vi "Enqueue Message.vi"(6 "Priority Message? (F)":bool=TRUE, 8 "error in (no error)":errorcluster, 10 "Message":T1={"Source"="", "Destination"="", "Time Stamp"=timestamp(0 s since 1904-01-01), "Command"="", "Data"=variant(string "")}, 11 "Listening Queue":refnum<queue>) -> (0 "error out":errorcluster, 3 "queue out":refnum<queue>)   [LabVIEW 2018, in "Dynamic Reentrant.lvlib"]
uses:
  <userlib>/Dynamic Reentrant/Dynamic Reentrant.lvlib
  <userlib>/Dynamic Reentrant/Type Defs/Message.ctl
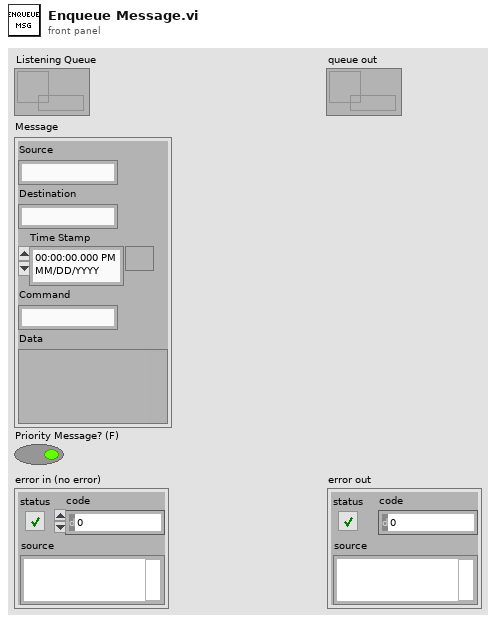
[diagram p1: front panel]
types:
  T1 = typedef "Dynamic Reentrant.lvlib/Message.ctl" = cluster{"Source":string, "Destination":string, "Time Stamp":timestamp, "Command":string, "Data":variant}
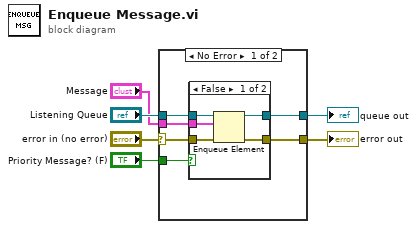
[diagram p0: block diagram]
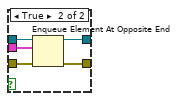
[diagram p2: hidden frame]
diagram:
  n1 = case shown="No Error" "error in (no error)" {
    selector: "error in (no error)" -> [w7 w23]
    tunnel: "Listening Queue" -> [w12 w24]
    tunnel: [w11 w23] -> w5
    tunnel: [w10 w24] -> w4
    tunnel: "Priority Message? (F)" -> [w9 _]
    tunnel: "Message" -> [w8 _]
    frame No Error {
      n2 = case shown="False" w9 {
        tunnel: w12 -> [w17 w22]
        tunnel: w7 -> [w16 w21]
        tunnel: [w15 w20] -> w11
        tunnel: [w14 w19] -> w10
        tunnel: w8 -> [w13 w18]
        frame False {
          n3 = Enqueue Element(queue=w17, element=w13, error in (no error)=w16) -> (queue out=w14:refnum<queue>, error out=w15:errorcluster)  [unwired: 1 in, 1 out]
        }
        frame True {
          n4 = Enqueue Element At Opposite End(queue=w22, element=w18, error in (no error)=w21) -> (queue out=w19:refnum<queue>, error out=w20:errorcluster)  [unwired: 1 in, 1 out]
        }
      }
    }
    frame Error {
    }
  }
  "error out" <- w5
  "queue out" <- w4
